vi "Launcher.vi"() -> (0 "error out":errorcluster)   [LabVIEW 2024]
uses:
  UI Actor/UI Actor/UI Actor/UI Actor.lvclass
  <vilib>/MGI/Panel Manager/Panel/Window Position/Reference Position/Alignment.ctl
  <vilib>/MGI/Panel Manager/Panel/Window Position/Reference Position/Horizontal Alignment.ctl
  <vilib>/MGI/Panel Manager/Panel/Window Position/Reference Position/Vertical Alignment.ctl
  <vilib>/MGI/Panel Manager/Panel/Window Position/Reference Position/Ref VI/Ref VI.lvclass
  <vilib>/MGI/Panel Manager/Panel/Window Position/Reference Position/Ref VI/Ref VI.vi
  <vilib>/MGI/Panel Manager/Panel Actor/Panel Actor/Launch Root Panel Window.vi
  <vilib>/MGI/Panel Manager/Panel Actor/Panel Actor/Panel Actor.lvclass
  <vilib>/MGI/Panel Manager/Panel/Panel.lvlib
  <vilib>/MGI/Panel Manager/Panel/Window Position/Reference Position/Reference Position.lvclass
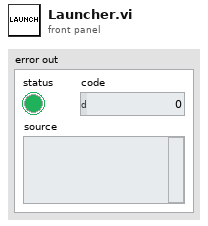
[diagram p1: front panel]
types:
  T1 = typedef "Panel.lvlib/Reference Position.lvclass/Alignment.ctl" = cluster{"Horizontal":T2, "Vertical":T3}
  T2 = typedef "Panel.lvlib/Reference Position.lvclass/Horizontal Alignment.ctl" = enum16{"Left", "Center", "Right"}
  T3 = typedef "Panel.lvlib/Reference Position.lvclass/Vertical Alignment.ctl" = enum16{"Top", "Center", "Bottom"}
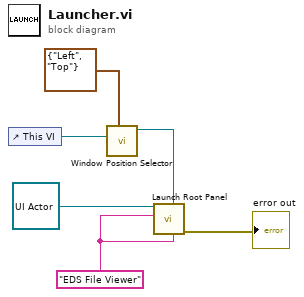
[diagram p0: block diagram]
diagram:
  w6 = "EDS File Viewer" ("Title")
  n1 = control-ref of="This VI"() -> (w2:refnum<vi>)
  n2 = call-poly <vilib>:"Window Position Selector.vi"("Alignment"=T1 {"Horizontal"=enum."Left", "Vertical"=enum."Top"}, "Ref VI"=w2) -> ("Ref VI out"=w3:refnum<class "Ref VI.lvclass">)  [unwired: 8 in, 1 out]
  n3 = call-poly <vilib>:"Launch Root Panel.vi"("Debug Alias"=w6, "Window Position (Maximize First Call)"=w3, "Title"=w6, "Panel Actor in"=refnum<class "UI Actor.lvclass"> refnum ("UI Actor.lvlib:UI Actor.lvclass")) -> ("Error Out"=→"error out":errorcluster)  [unwired: 6 in, 1 out]
